vi "Disabled.vi"(7 "Robot Mode":T3, 10 "Match Info":T2={"Autonomous Elapsed Seconds"=0.0, "TeleOp Elapsed Seconds"=0.0, "Disabled Elapsed Seconds"=0.0, "Visited Autonomous"=FALSE, "Visited TeleOp"=FALSE, "Visited Disabled"=FALSE, "Autonomous Settings"={"Autonomous Style"=enum."Independent", "VI Refnum"=refnum}}, 11 "Call Context":T1) -> ()   [LabVIEW 2020]
doc: "This VI is called each time a disabled packet is received from the DS. It can be used to prepare for the next robot mode, to calibrate sensors, etc."
uses:
  <vilib>/Rock Robotics/WPI/DriverStation/WPI_DriverStationRobotMode2.ctl
  <vilib>/Rock Robotics/WPI/DriverStation/WPI_DriverStationMatch Info.ctl
  <vilib>/Rock Robotics/WPI/DriverStation/WPI_DriverStationDerivedRobotMode.ctl
  <vilib>/Rock Robotics/Network Tables/NT Read Boolean.vi
  <vilib>/Rock Robotics/Network Tables/NT Write Number.vi
  Drive/Implementation/Infrastructure/Drive Command Helper.vi
  f24b0b83-2279-442d-80fd-e43a507541fa.vi
  926d9f57-6829-42fd-b42e-84e2e012e831.vi
panel:
  in  "Numeric":dbl=1.0 format="%#_13g"
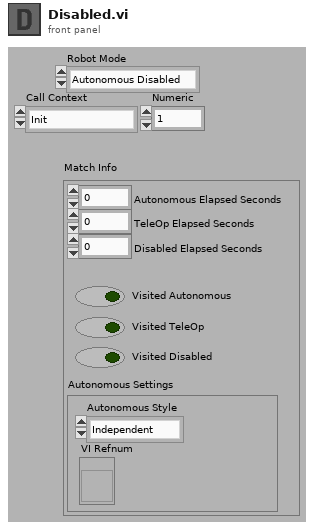
[diagram p1: front panel]
types:
  T1 = typedef "WPI_DriverStationDerivedRobotMode.ctl" = enum16{"Init", "Execute", "Stop"}
  T2 = typedef "WPI_DriverStationMatch Info.ctl" = cluster{"Autonomous Elapsed Seconds":dbl, "TeleOp Elapsed Seconds":dbl, "Disabled Elapsed Seconds":dbl, "Visited Autonomous":bool, "Visited TeleOp":bool, "Visited Disabled":bool, "Autonomous Settings":cluster{"Autonomous Style":enum16{"Iterative", "Independent"}, "VI Refnum":refnum<vi>}}
  T3 = typedef "WPI_DriverStationRobotMode2.ctl" = enum16{"Autonomous Disabled", "Autonomous Enabled", "Teleop Disabled", "Teleop Enabled", "Disconnected", "Finish", "Test Disabled", "Test Enabled", "Emergency Stopped"}
  T4 = typedef "ADIS16470 Device Reference.ctl" = cluster{"DevStatus":errorcluster, "Hardware Config":T5, "Calibration Complete":refnum<notifier>, "Status Reference":refnum<data-value>, "Position Reference":refnum<data-value>, "Velocity Reference":refnum<data-value>, "Sychronous Process VI":T9, "Cmd FIFO":refnum<k33>, "Source":T10, "Data FIFO":refnum<k33>, "Calibration Time (ms)":u32}
  T5 = typedef "ADIS16470 Hardware Configuration.ctl" = cluster{"SPI Clock Rate (Hz)":dbl, "IMU SPI Mode (3)":T6, "IMU Reset Pin":T7, "IMU SPI Bus":T8, "IMU Data Ready Pin":T7, "Stall Config":cluster{"Pow2BytesPerRead":u8, "StallTicks":u16, "CsToSclkTicks":u8}}
  T6 = typedef "WPI_SPIMode.ctl" = enum16{"Mode 0 (Clk Idle Low,Sample on Leading)", "Mode 1 (Clk Idle Low,Sample on Trailing)", "Mode 2 (Clk Idle High,Sample on Leading)", "Mode 3 (Clk Idle High,Sample on Trailing)"}
  T7 = typedef "FPGA_DIOChannel.ctl" = enum8{"DIO 0", "DIO 1", "DIO 2", "DIO 3", "DIO 4", "DIO 5", "DIO 6", "DIO 7", "DIO 8", "DIO 9", "DIO MXP 0", "DIO MXP 1", "DIO MXP 2", "DIO MXP 3", "DIO MXP 4", "DIO MXP 5", "DIO MXP 6", "DIO MXP 7", "DIO MXP 8", "DIO MXP 9", "DIO MXP 10", "DIO MXP 11", "DIO MXP 12", "DIO MXP 13", "DIO MXP 14", "DIO MXP 15", "SPI Port CS1", "SPI Port CS2", "SPI Port CS3", "SPI Port MISO", "SPI Port MOSI", "Invalid"}
  T8 = typedef "spi_bus.ctl" = enum16{"SPI On-Board, CS0", "SPI On-Board, CS1", "SPI On-Board, CS2", "SPI On-Board, CS3", "SPI MXP", "Invalid"}
  T9 = typedef "ADIS16470 Process.ctl" = refnum<vi>
  T10 = typedef "FPGA_CounterEncoderSourceConvertionLVSourceType.ctl" = cluster{"DevStatus":errorcluster, "AnalogTriggerMode?":bool, "DigitalMode":cluster{"DIO Channel":T11}, "AnalogTriggerMode":cluster{"AnalogTriggerIndex":T12, "OutputType":T13}}
  T11 = typedef "FPGA_DIODigitalSourceChannel.ctl" = enum8{"DIO 0", "DIO 1", "DIO 2", "DIO 3", "DIO 4", "DIO 5", "DIO 6", "DIO 7", "DIO 8", "DIO 9", "DIO MXP 0", "DIO MXP 1", "DIO MXP 2", "DIO MXP 3", "DIO MXP 4", "DIO MXP 5", "DIO MXP 6", "DIO MXP 7", "DIO MXP 8", "DIO MXP 9", "DIO MXP 10", "DIO MXP 11", "DIO MXP 12", "DIO MXP 13", "DIO MXP 14", "DIO MXP 15", "SPI Port CS1", "SPI Port CS2", "SPI Port CS3", "SPI Port MISO", "SPI Port MOSI", "Disabled"}
  T12 = typedef "FPGA_AnalogTriggerIndex.ctl" = enum8{"Trig 0", "Trig 1", "Trig 2", "Trig 3", "Trig 4", "Trig 5", "Trig 6", "Trig 7", "Invalid"}
  T13 = typedef "FPGA_AnalogTriggerOutType.ctl" = enum16{"InWindow", "TriggerState", "Rising", "Falling"}
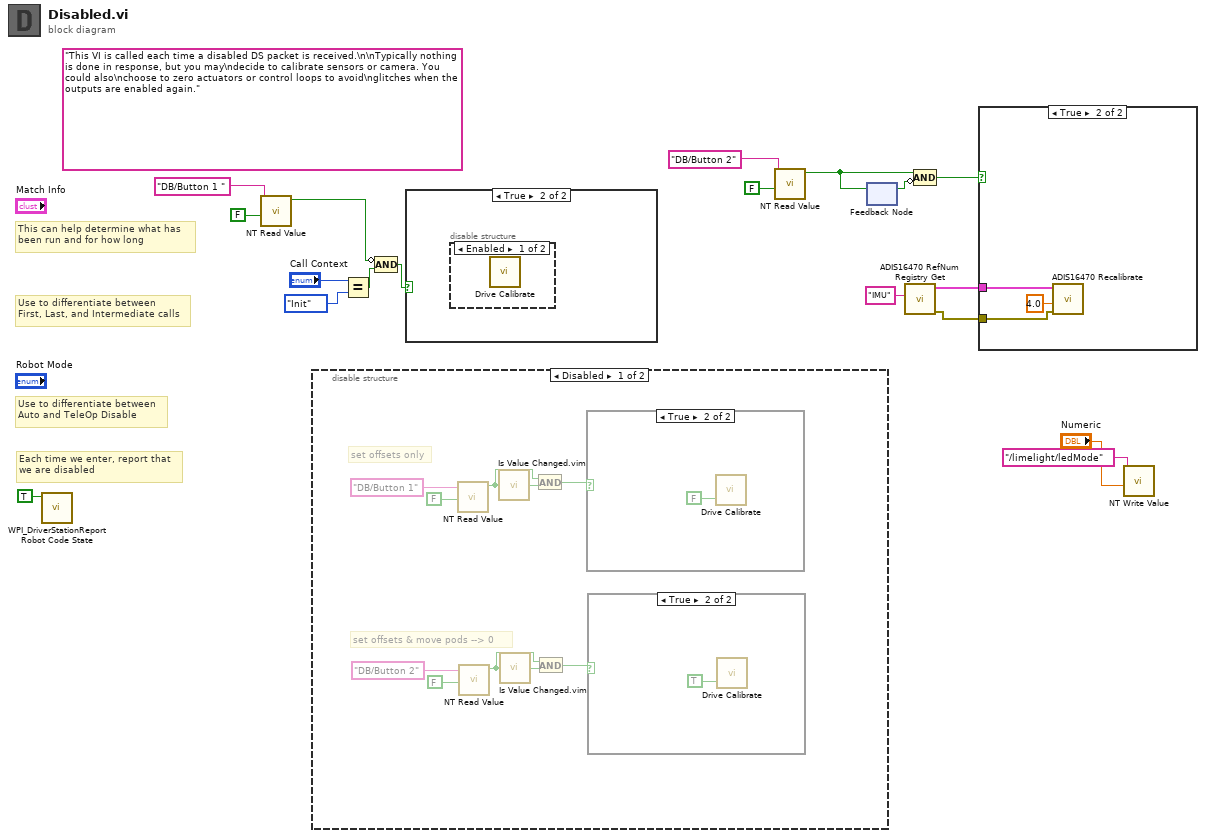
[diagram p0: block diagram]
diagram:
  (unwired) "This VI is called each time a disabled DS packet is received.\n\nTypically nothing is done in response, but you may\ndecide to calibrate sensors or camera. You could also\nchoose to zero actuators or control loops to avoid\nglitches when the outputs are enabled again."
  # "Each time we enter, report that\nwe are disabled"
  # "Use to differentiate between\nFirst, Last, and Intermediate calls"
  # "This can help determine what has\nbeen run and for how long"
  # "Use to differentiate between\nAuto and TeleOp Disable"
  n1 = call <vilib>:"WPI_DriverStationReport Robot Code State.vi"("Disabled"=TRUE ("Autonomous")) -> ()  [unwired: 10 in, 1 out]
  n2 = call-poly <vilib>:"NT Read Value.vi"("Default Value"=FALSE, "Name"="DB/Button 1 ") -> ("Boolean"=w12:bool)  [unwired: 8 in, 1 out]
  n3 = disable-structure shown="Disabled" {
    frame Disabled {
      # "set offsets only"
      # "set offsets & move pods --> 0"
      n4 = call-poly <vilib>:"NT Read Value.vi"("Default Value"=FALSE, "Name"="DB/Button 1") -> ("Boolean"=w24:bool)  [unwired: 8 in, 1 out]
      n5 = call-poly <vilib>:"NT Read Value.vi"("Default Value"=FALSE, "Name"="DB/Button 2") -> ("Boolean"=w23:bool)  [unwired: 8 in, 1 out]
      n6 = call "Is Value Changed.vim"("value"=w24) -> ("changed or first call?"=w25:bool)
      n7 = call "Is Value Changed.vim"("value"=w23) -> ("changed or first call?"=w22:bool)
      n8 = And(x=w24, y=w25) -> (x .and. y?=w26:bool)
      n9 = And(x=w23, y=w22) -> (x .and. y?=w21:bool)
      n10 = case shown="True" w26 {
        frame False {
        }
        frame True {
          n11 = call "Drive Calibrate.vi"("reset pods"=FALSE) -> ()  [unwired: 10 in, 1 out]
        }
      }
      n12 = case shown="True" w21 {
        frame False {
        }
        frame True {
          n13 = call "Drive Calibrate.vi"("reset pods"=TRUE) -> ()  [unwired: 10 in, 1 out]
        }
      }
    }
    frame Enabled {
    }
  }
  n14 = Equal?(x="Call Context", y=WPI_DriverStationDerivedRobotMode."Init") -> (x = y?=w13:bool)
  n15 = Compound Arithmetic op=AND(invert w12, w13) -> (w11:bool)
  n16 = case shown="True" w11 {
    frame False {
    }
    frame True {
      n17 = disable-structure shown="Enabled" {
        frame Enabled {
          n18 = call "Drive Calibrate.vi"() -> ()  [unwired: 11 in, 1 out]
        }
        frame Disabled {
        }
      }
    }
  }
  n19 = call-poly <vilib>:"NT Read Value.vi"("Default Value"=FALSE, "Name"="DB/Button 2") -> ("Boolean"=w7:bool)  [unwired: 8 in, 1 out]
  n20 = feedback-in #1(w7) -> ()
  n21 = feedback #1() -> (w8:bool)  [unwired: 1 in]
  n22 = call "ADIS16470 RefNum Registry Get.vi"("refnum name"="IMU") -> ("error out"=w3:errorcluster, "ADIS16470DevRef out"=w4:T4)  [unwired: 9 in]
  n23 = Compound Arithmetic op=AND(w7, invert w8) -> (w6:bool)
  n24 = case shown="True" w6 {
    tunnel: w4 -> [_ w32]
    tunnel: w3 -> [_ w31]
    frame False {
    }
    frame True {
      n25 = call "ADIS16470 Recalibrate.vi"("error in (no error)"=w31, "Calibration Time (4s)"=4.0, "ADIS16470DevRef in"=w32) -> ()  [unwired: 7 in, 2 out]
    }
  }
  n26 = call-poly <vilib>:"NT Write Value.vi"("Numeric"="Numeric", "Name"="/limelight/ledMode") -> ()  [unwired: 9 in, 1 out]
